vi "Destroy Message-Enqueuer References VI Name.vi"() -> (0 "Destroy Message Enqueue References VI":string="Create Message Enqueue References.vi")   [LabVIEW 2018, in "Scripting.lvlib"]
uses:
  Scripting.lvlib
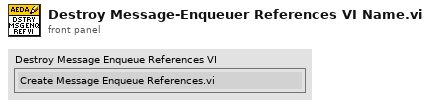
[diagram p1: front panel]
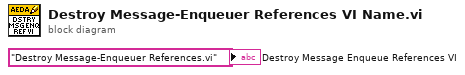
[diagram p0: block diagram]
diagram:
  "Destroy Message Enqueue References VI" <- "Destroy Message-Enqueuer References.vi"
